vi "Takktile_LabView.vi"() -> ()   [LabVIEW 2011]
uses:
  <vilib>/Instr/_visa.llb/VISA Set IO Buffer Mask.ctl
  <vilib>/Instr/_visa.llb/VISA Configure Serial Port (Instr).vi
panel:
  in  "Select Serial Port":refnum<visa-resource-name>="COM3"
  in  "Offset":bool
  out "Bytes remaining at SP":u32
  out "Takktile Measurements":dbl[](array[slide])=[229.0, 89.0, 105.0, 116.0, 139.0, 201.0, 194.0, 112.0, 143.0, 164.0] scale=-50.0..700.0
  in  "byte size for buffer":u32=200
  out "error out":errorcluster
  in  "stop":bool
  out "bytes readint":u32=92
  out "Takktile Reading":string="[371.00],[511.00],[495.00],[484.00],[461.00],[399.00],[406.00],[488.00],[457.00],[436.00]]\r\n"
  # "1. Select Serial Port at which the sensors are streaming data\n2. If you have more sensors than currently displaying at the graph, drag the matrix right. \n3. Run the VI\n4. Press Offset to set the zero reading at the current force level for all sensors"
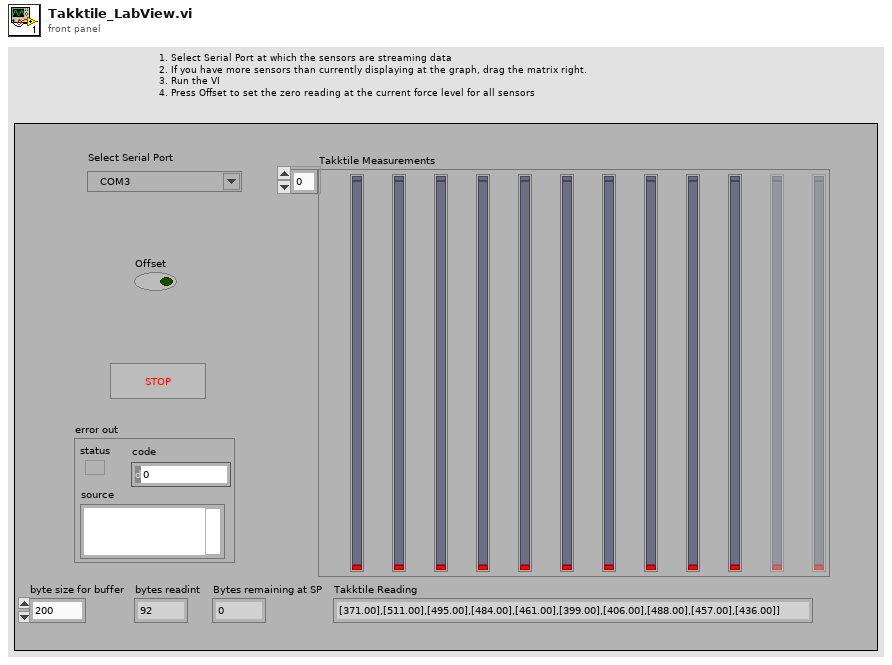
[diagram p1: front panel]
types:
  T1 = typedef "VISA Set IO Buffer Mask.ctl" = u16
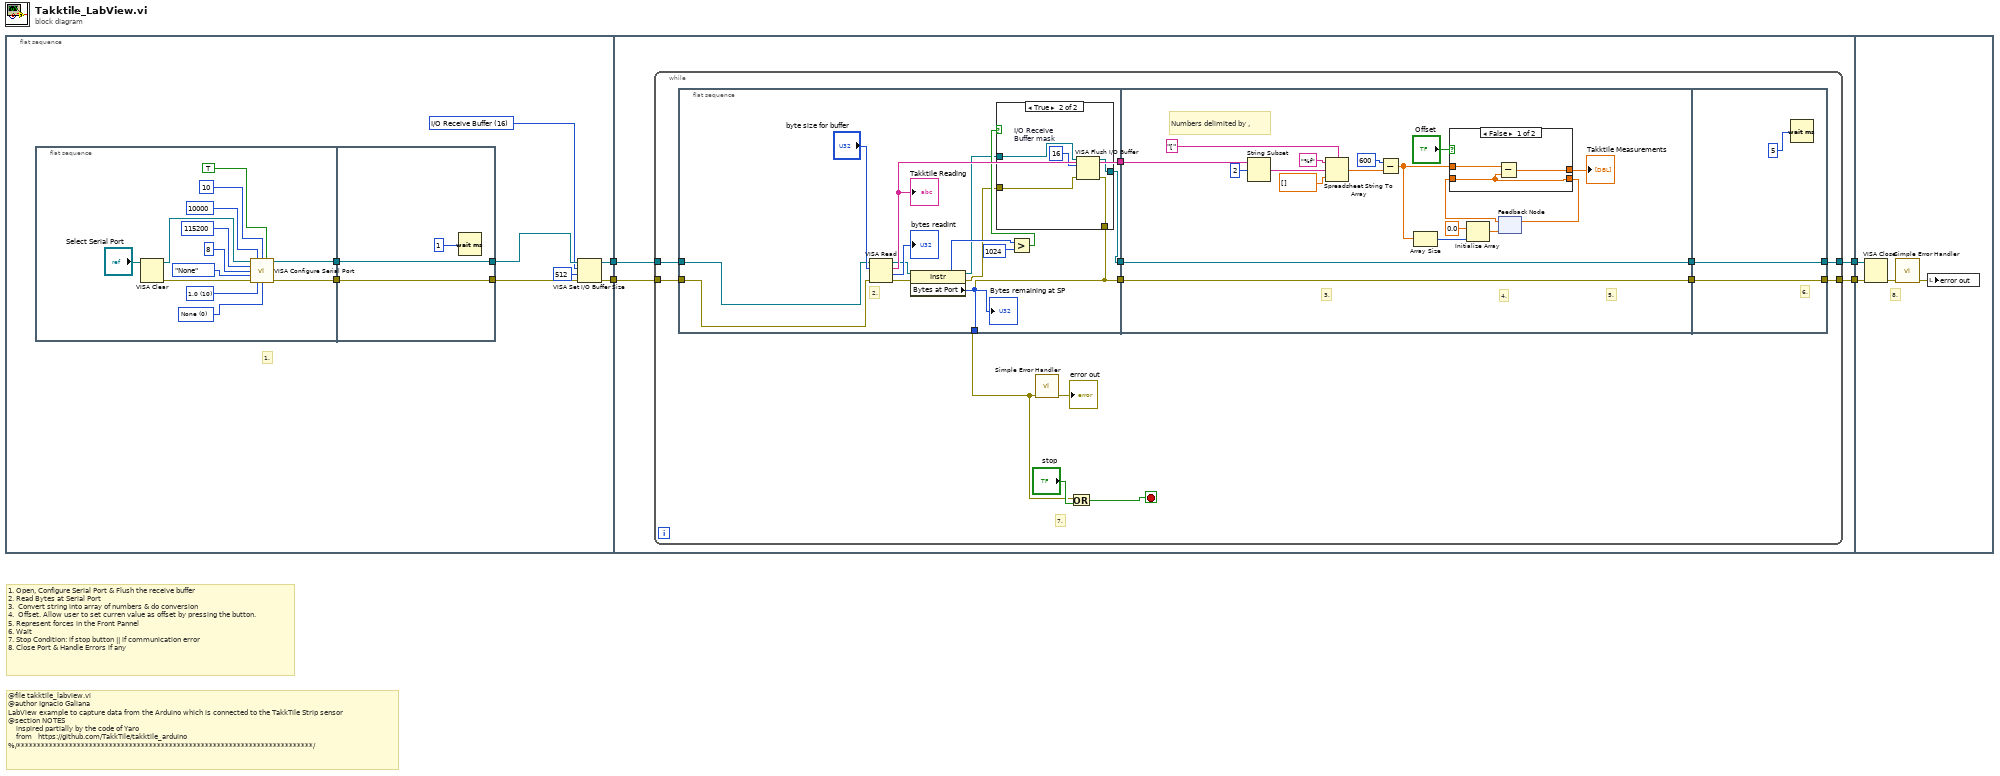
[diagram p0: block diagram]
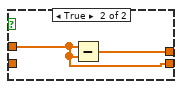
[diagram p3: hidden frame]
diagram:
  # "@file takktile_labview.vi\n@author Ignacio Galiana\nLabView example to capture data from the Arduino which is connected to the TakkTile Strip sensor\n@section NOTES\n    inspired partially by the code of Yaro\n    from   https://github.com/TakkTile/takktile_arduino\n%/**************************************************************************/"
  # "1. Open, Configure Serial Port & Flush the receive buffer\n2. Read Bytes at Serial Port\n3.  Convert string into array of numbers & do conversion\n4.  Offset. Allow user to set curren value as offset by pressing the button.\n5. Represent forces in the Front Pannel\n6. Wait\n7. Stop Condition: if stop button || if communication error\n8. Close Port & Handle Errors if any"
  n1 = flat-sequence {
    tunnel: [w8] -> w4
    tunnel: [w7] -> w3
    tunnel: [w32] -> w2
    tunnel: [w31] -> w1
    tunnel: w4 -> [w29]
    tunnel: w3 -> [w30]
    tunnel: w2 -> [w96]
    tunnel: w1 -> [w95]
    frame #0 {
      w6 = T1 16 items=["I/O Receive Buffer"=16, "I/O Transmit Buffer"=32, "I/O Receive and Transmit Buffer"=48] ("Mask")
      # "1."
      n2 = flat-sequence {
        tunnel: [w14] -> w12
        tunnel: [w13] -> w11
        tunnel: [w27] -> w9
        tunnel: [w28] -> w10
        tunnel: w12 -> [w28]
        tunnel: w11 -> [w27]
        frame #0 {
          w19 = u16 10 items=["1.0"=10, "1.5"=15, "2.0"=20] ("stop bits (10: 1 bit)")
          w22 = u16 0 items=["None", "XON/XOFF", "RTS/CTS", "XON/XOFF & RTS/CTS", "DTR/DSR", "XON/XOFF & DTR/DSR"] ("flow control (0:none)")
          n3 = VISA Clear(VISA resource name="Select Serial Port") -> (VISA resource name out=w16:refnum<visa-resource-name>, error out=w15:errorcluster)  [unwired: 1 in]
          n4 = call-poly "VISA Configure Serial Port"("VISA resource name"=w16, "timeout (10sec)"=u32 10000, "termination char\n(0xA = '\\n' = LF)"=u8 10 ("termination char\n(0xA = '\\n' = LF)"), "Enable Termination\nChar (T)"=TRUE ("Enable Termination\nChar (T)"), "baud rate (9600)"=u32 115200, "data bits (8)"=u16 8, "parity (0:none)"=enum16{"None", "Odd", "Even", "Mark", "Space"}."None", "error in (no error)"=w15, "stop bits (10: 1 bit)"=w19, "flow control (0:none)"=w22) -> ("VISA resource name out"=w14:refnum<visa-resource-name>, "error out"=w13:errorcluster)  [unwired: 4 in]
        }
        frame #1 {
          n5 = Wait (ms)(milliseconds to wait=u32 1 ("milliseconds to wait 2")) -> ()  [unwired: 1 out]
        }
      }
      n6 = VISA Set I/O Buffer Size(VISA resource name=w10, mask (16)=w6, size (4096)=u32 512, error in (no error)=w9) -> (VISA resource name out=w7:refnum<visa-resource-name>, error out=w8:errorcluster)
    }
    frame #1 {
      n7 = while {
        tunnel: [w45] -> w32
        tunnel: [w44] -> w31
        tunnel: w30 -> [w40]
        tunnel: w29 -> [w39]
        stop <- w33 stop-if-true
        # "7."
        n8 = flat-sequence {
          tunnel: w39 -> [w53]
          tunnel: [w46] -> w43
          tunnel: [w47] -> w42
          tunnel: w40 -> [w54]
          tunnel: [w46] -> w35
          tunnel: [w51] -> _
          tunnel: [w57] -> w38
          tunnel: w43 -> [w83]
          tunnel: w42 -> [w84]
          tunnel: w38 -> [w77]
          tunnel: [w84] -> w37
          tunnel: [w83] -> w36
          tunnel: [w91] -> w44
          tunnel: [w92] -> w45
          tunnel: w37 -> [w92]
          tunnel: w36 -> [w91]
          frame #0 {
            # "2."
            n9 = VISA Read(VISA resource name=w54, byte count="byte size for buffer", error in (no error)=w53) -> (VISA resource name out=w56:refnum<visa-resource-name>, read buffer=w57:string, return count=→"bytes readint":u32, error out=w55:errorcluster)
            "Takktile Reading" <- w57
            n10 = property class="Instr"(reference=w56, error in=w55) -> (reference out=w49:refnum<visa-resource-name>, error out=w48:errorcluster, "Bytes at Port"=w51:u32)
            "Bytes remaining at SP" <- w51
            n11 = Greater?(x=w51, y=u32 1024) -> (0:w50:bool)
            n12 = case shown="True" w50 {
              tunnel: w49 -> [w61 w65]
              tunnel: w48 -> [w60 w64]
              tunnel: [w61 w63] -> w47
              tunnel: [w60 w62] -> w46
              frame False {
              }
              frame True {
                w66 = u16 16  # I/O Receive Buffer mask
                n13 = VISA Flush I/O Buffer(VISA resource name=w65, mask (16)=w66, error in (no error)=w64) -> (VISA resource name out=w63:refnum<visa-resource-name>, error out=w62:errorcluster)
              }
            }
          }
          frame #1 {
            # "5."
            # "Numbers delimited by ,"
            # "3."
            # "4."
            n14 = String Subset(string=w77, offset (0)=2) -> (substring=w75:string)  [unwired: 1 in]
            n15 = Spreadsheet String To Array(delimiter (Tab)="[", format string="%f", spreadsheet string=w75, array type (2D Dbl)=dbl[] []) -> (array=w73:dbl[])
            n16 = Subtract(x=u32 600 ("y"), y=w73) -> (x-y=w71:dbl[])
            n17 = Array Size(array=w71) -> (size(s)=w70:i32)
            n18 = Initialize Array(0.0 ("element"), w70) -> (w68:dbl[])
            n19 = feedback #1(w68) -> (w80:dbl[])
            n20 = case shown="False" "Offset" {
              tunnel: w71 -> [w86 w88]
              tunnel: [w87 w89] -> w67
              tunnel: [w85 w88] -> w81
              tunnel: w80 -> [w85 _]
              frame False {
                n21 = Subtract(x=w86, y=w85) -> (x-y=w87:dbl[])
              }
              frame True {
                n22 = Subtract(x=w88, y=w88) -> (x-y=w89:dbl[])
              }
            }
            "Takktile Measurements" <- w67
            n23 = feedback-in #1(w81) -> ()
          }
          frame #2 {
            # "6."
            n24 = Wait (ms)(milliseconds to wait=u32 5) -> ()  [unwired: 1 out]
          }
        }
        n25 = call <vilib>:"Simple Error Handler.vi"("error in (no error)"=w35) -> ("error out"=→"error out":errorcluster)  [unwired: 4 in, 4 out]
        n26 = Or(x=w35, y="stop") -> (x .or. y?=w33:bool)
      }
    }
    frame #2 {
      # "8."
      n27 = VISA Close(VISA resource name=w96, error in (no error)=w95) -> (error out=w94:errorcluster)
      n28 = call <vilib>:"Simple Error Handler.vi"("error in (no error)"=w94) -> ("error out"=w93:errorcluster)  [unwired: 4 in, 4 out]
      n29 = local write "error out"(w93) -> ()
    }
  }
